vi "trash_Fix Plugin UI Dependencies.vi"(8 "error in":errorcluster, 10 "Project Path":path, 11 "VI Refnum in":refnum<vi>) -> (0 "error out":errorcluster, 3 "VI Refnum out":refnum<vi>)   [LabVIEW 2021]
uses:
  <vilib>/Utility/traverseref.llb/TRef TravTarget.ctl
  <vilib>/Utility/traverseref.llb/VI Scripting - Traverse.lvlib
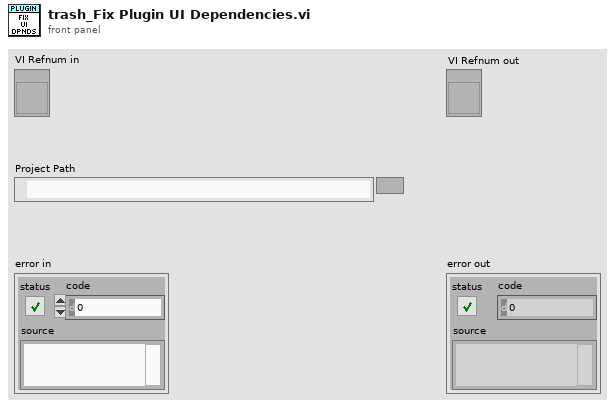
[diagram p1: front panel]
types:
  T1 = typedef "TRef TravTarget.ctl" = enum16{"FP", "BD", "Other"}
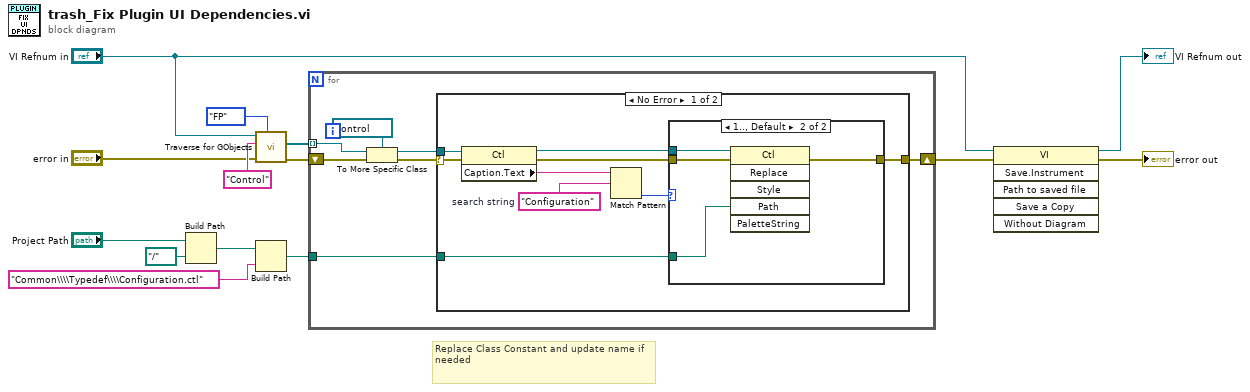
[diagram p0: block diagram]
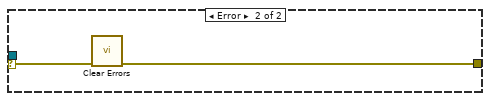
[diagram p3: hidden frame]
diagram:
  # "Replace Class Constant and update name if needed"
  n1 = Build Path(base path="Project Path", name or relative path=path "../..") -> (appended path=w9:path)
  n2 = call <vilib>:"Traverse for GObjects.vi"("Traverse Target"=TRef_TravTarget."FP", "error in (no error)"="error in", "Class Name"="Control", "VI Refnum"="VI Refnum in") -> ("error out"=w7:errorcluster, "References"=w13:refnum<vi>[])  [unwired: 4 in, 2 out]
  n3 = Build Path(base path=w9, name or relative path="Common\\\\Typedef\\\\Configuration.ctl" ("Class Name")) -> (appended path=w6:path)
  n4 = for {
    tunnel: w13 -> [w21] mode=indexing
    shift-right: [w19] -> w3
    shift-left: w7 -> [w17]
    tunnel: w6 -> [w16]
    n5 = To More Specific Class(target class=refnum<vi> refnum ("x"), reference=w21, error in=w17) -> (specific class reference=w18:refnum<vi>, error out=w15:errorcluster)
    n6 = case shown="No Error" w15 {
      selector: w15 -> [w22 w37]
      tunnel: [w28 w36] -> w19
      tunnel: w18 -> [w27 _]
      tunnel: w16 -> [w25 _]
      frame No Error {
        w24 = "Configuration"  # search string
        n7 = property class="Ctl"(reference=w27, error in=w22) -> (reference out=w29:refnum<vi>, error out=w30:errorcluster, "Caption.Text"=w26:string)
        n8 = Match Pattern(string=w26, regular expression=w24) -> (offset past match=w23:i32)  [unwired: 1 in, 3 out]
        n9 = case shown="1.., Default" w23 {
          tunnel: w30 -> [w31 w33]
          tunnel: w29 -> [_ w32]
          tunnel: [w31 w35] -> w28
          tunnel: w25 -> [_ w34]
          frame -1 {
          }
          frame 1.., Default {
            n10 = invoke class="Ctl" method="Replace"(reference=w32, error in=w33, "Path"=w34) -> (error out=w35:errorcluster)  [unwired: 3 in, 5 out]
          }
        }
      }
      frame Error {
        n11 = call <vilib>:"Clear Errors.vi"("error in (no error)"=w37) -> ("error out"=w36:errorcluster)  [unwired: 5 in, 1 out]
      }
    }
  }
  n12 = invoke class="VI" method="Save.Instrument"(reference="VI Refnum in", error in=w3) -> (reference out=→"VI Refnum out":refnum<vi>, error out=→"error out":errorcluster)  [unwired: 4 in, 4 out]
